vi "MGI Rotate Vector (SGL).vi"(1 "Right Hand Rotation":sgl format="%.2f", 2 "Rotation Axis":T1, 3 "Input Vector":sgl[](array[numeric]) format="%.2f") -> (0 "Rotated Vector":sgl[](array[numeric]) format="%.2f")   [LabVIEW 2016]
doc: "Perform a 3D vector rotation about a coordinate axis.\n\nAuthored by David A. Moore\nsupport@mooregoodideas.com\nwww.mooregoodideas.com\n\nCopyright (c) 2010, Moore Good Ideas, Inc.\n\nAll rights reserved.\n\nRedistribution and use in source and binary forms, with or without modification, are permitted provided that the following conditions are met:\n\n * Redistributions of source code must retain the above copyright notice, this list of conditions and the following disclaimer.\n * Redistributions in binary form must reproduce the above copyright notice, this list of conditions and the following disclaimer in the documentation and/or other materials provided with the distribution.\n * Neither the name of Moore Good Ideas, Inc. nor the names of its contributors may be used to endorse or promote products derived from this software without specific prior written permission.\n\nTHIS SOFTWARE IS PROVIDED BY THE COPYRIGHT HOLDERS AND CONTRIBUTORS \"AS IS\" AND ANY EXPRESS OR IMPLIED WARRANTIES, INCLUDING, BUT NOT LIMITED TO, THE IMPLIED WARRANTIES OF MERCHANTABILITY AND FITNESS FOR A PARTICULAR PURPOSE ARE DISCLAIMED. IN NO EVENT SHALL THE COPYRIGHT OWNER OR CONTRIBUTORS BE LIABLE FOR ANY DIRECT, INDIRECT, INCIDENTAL, SPECIAL, EXEMPLARY, OR CONSEQUENTIAL DAMAGES (INCLUDING, BUT NOT LIMITED TO, PROCUREMENT OF SUBSTITUTE GOODS OR SERVICES; LOSS OF USE, DATA, OR PROFITS; OR BUSINESS INTERRUPTION) HOWEVER CAUSED AND ON ANY THEORY OF LIABILITY, WHETHER IN CONTRACT, STRICT LIABILITY, OR TORT (INCLUDING NEGLIGENCE OR OTHERWISE) ARISING IN ANY WAY OUT OF THE USE OF THIS SOFTWARE, EVEN IF ADVISED OF THE POSSIBILITY OF SUCH DAMAGE.."
uses:
  <userlib>/_MGI/Coordinates/MGI Coordinate Axis Enum.ctl
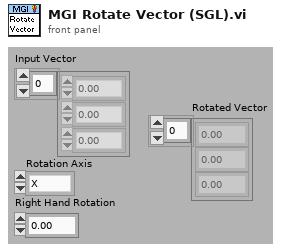
[diagram p1: front panel]
types:
  T1 = typedef "MGI Coordinate Axis Enum.ctl" = enum16{"X", "Y", "Z"}
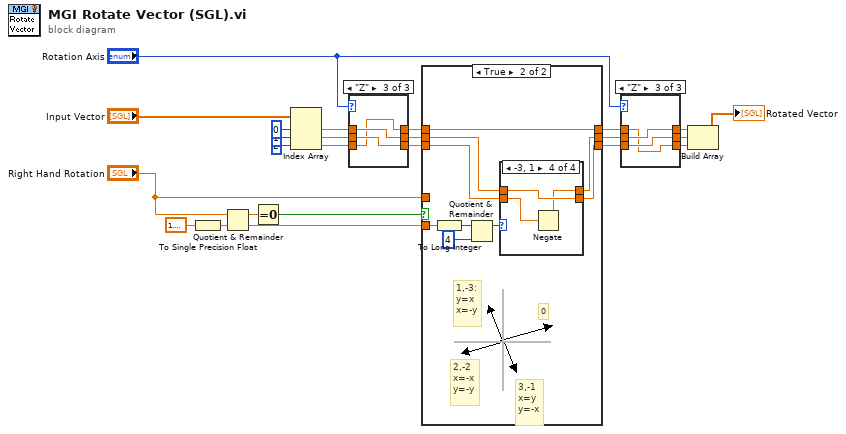
[diagram p0: block diagram]
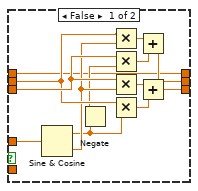
[diagram p2: hidden frame]
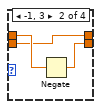
[diagram p4: hidden frame]
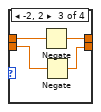
[diagram p5: hidden frame]
diagram:
  n1 = To Single Precision Float(number=1.5707963267948966) -> (single precision float=w5:sgl)
  n2 = Quotient & Remainder(x="Right Hand Rotation", y=w5) -> (x-y*floor(x/y)=w24:sgl, floor(x/y)=w7:sgl)
  n3 = Equal To 0?(x=w24) -> (x = 0?=w8:bool)
  n4 = Index Array(array="Input Vector", index #1=0 ("Index"), index #2=1 ("Index"), index #3=2 ("Index")) -> (element #1=w20:sgl, element #2=w19:sgl, element #3=w18:sgl)
  n5 = case shown="\"Z\"" "Rotation Axis" {
    tunnel: [w27 w30 w31] -> w10
    tunnel: w20 -> [w27 w28 w32]
    tunnel: [w26 w29 w32] -> w11
    tunnel: w19 -> [w26 w30 w33]
    tunnel: [w25 w28 w33] -> w12
    tunnel: w18 -> [w25 w29 w31]
    frame "X" {
    }
    frame "Y" {
    }
    frame "Z" {
    }
  }
  n6 = case shown="True" w8 {
    tunnel: "Right Hand Rotation" -> [w46 _]
    tunnel: [w45 w47] -> w14
    tunnel: [w40 w48] -> w13
    tunnel: w12 -> [w39 w49]
    tunnel: w11 -> [w38 w50]
    tunnel: w10 -> [w34 w54]
    tunnel: [w34 w54] -> w9
    tunnel: w7 -> [_ w55]
    frame False {
      n7 = Sine & Cosine(0:w46) -> (1:w36:sgl, 2:w37:sgl)
      n8 = Negate(x=w36) -> (-x=w35:sgl)
      n9 = Multiply(x=w38, y=w37) -> (x*y=w41:sgl)
      n10 = Multiply(x=w39, y=w35) -> (x*y=w42:sgl)
      n11 = Multiply(x=w39, y=w37) -> (x*y=w44:sgl)
      n12 = Multiply(x=w38, y=w36) -> (x*y=w43:sgl)
      n13 = Add(x=w41, y=w42) -> (x+y=w40:sgl)
      n14 = Add(x=w44, y=w43) -> (x+y=w45:sgl)
    }
    frame True {
      # "3,-1\nx=y\ny=-x"
      # "2,-2\nx=-x\ny=-y"
      # "1,-3:\ny=x\nx=-y"
      # "0"
      n15 = To Long Integer(number=w55) -> (32bit integer=w53:i32)
      n16 = Quotient & Remainder(x=w53, y=4) -> (x-y*floor(x/y)=w51:i32)  [unwired: 1 out]
      n17 = case shown="-3, 1" w51 {
        tunnel: w50 -> [w57 w60 w64 w66]
        tunnel: w49 -> [w56 w58 w62 w67]
        tunnel: [w57 w58 w63 w65] -> w48
        tunnel: [w56 w59 w61 w66] -> w47
        frame ..-4, 0, 4.. {
        }
        frame -1, 3 {
          n18 = Negate(x=w60) -> (-x=w59:sgl)
        }
        frame -2, 2 {
          n19 = Negate(x=w64) -> (-x=w63:sgl)
          n20 = Negate(x=w62) -> (-x=w61:sgl)
        }
        frame -3, 1 {
          n21 = Negate(x=w67) -> (-x=w65:sgl)
        }
      }
    }
  }
  n22 = case shown="\"Z\"" "Rotation Axis" {
    tunnel: [w70 w71 w76] -> w17
    tunnel: w9 -> [w70 w72 w74]
    tunnel: [w69 w72 w75] -> w16
    tunnel: w13 -> [w69 w73 w76]
    tunnel: [w68 w73 w74] -> w15
    tunnel: w14 -> [w68 w71 w75]
    frame "X" {
    }
    frame "Y" {
    }
    frame "Z" {
    }
  }
  n23 = Build Array(w17, w16, w15) -> (→"Rotated Vector":sgl[])
